vi "Is Msg.vi"(9 "Msg":refnum<class "Msg.lvclass">, 10 "Msgs":T1) -> (2 "Error":errorcluster)   [LabVIEW 2020, in "jettl.lvlib" / "Actor.lvlib"]
uses:
  Actor.lvlib
  Msgs.ctl
  Msg/Msg.lvclass
  Error/Error.lvlib
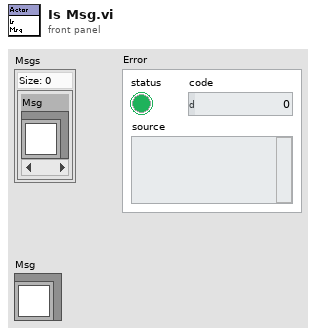
[diagram p1: front panel]
types:
  T1 = typedef "jettl.lvlib/Actor.lvlib/Msgs.ctl" = set{refnum<class "Msg.lvclass">}
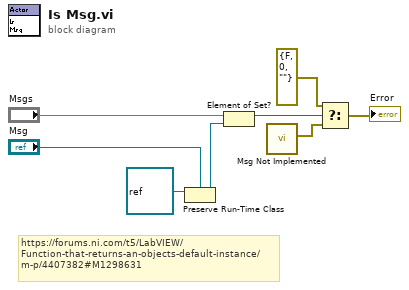
[diagram p0: block diagram]
diagram:
  # "https://forums.ni.com/t5/LabVIEW/Function-that-returns-an-objects-default-instance/m-p/4407382#M1298631"
  n1 = Preserve Run-Time Class(object in=refnum<class> refnum ("LabVIEW Object"), 2:"Msg") -> (object out=w8:refnum<class "Msg.lvclass">)  [unwired: 1 in, 1 out]
  n2 = Element of Set?(10:w8, 11:"Msgs") -> (3:w2:bool)
  n3 = call "Msg Not Implemented.vi"() -> ("Error"=w3:errorcluster)  [unwired: 11 in]
  n4 = Select(t=errorcluster {"status"=FALSE, "code"=0, "source"=""} ("Error"), s=w2, f=w3) -> (s? t:f=→"Error":errorcluster)
